vi "Pid_v00.vi"() -> ()   [LabVIEW 2010]
panel:
  in  "stop":bool
  out "u,y,r":cluster{"y":dbl, "u":dbl, "r-Set point":dbl}(graph)={"y"=50.04611274315553, "u"=50.10510244223579, "r-Set point"=50.0}
  in  "Kd":dbl(slide)=0.1151685393258427 scale=0.0..0.5
  in  "Ki":dbl(slide)=0.8764044943820224 scale=0.0..2.0
  in  "Kp":dbl(slide)=0.33707865168539325 scale=0.0..2.5
  out "y-Iesirea":dbl(slide)=50.04611274315553 scale=40.0..60.0
  out "u":dbl(slide)=50.10510244223579 scale=40.0..60.0
  in  "r-Set point":dbl(slide)=50.0 scale=40.0..60.0
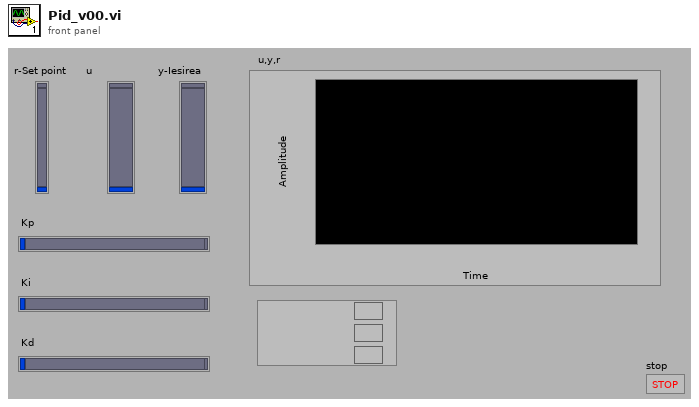
[diagram p1: front panel]
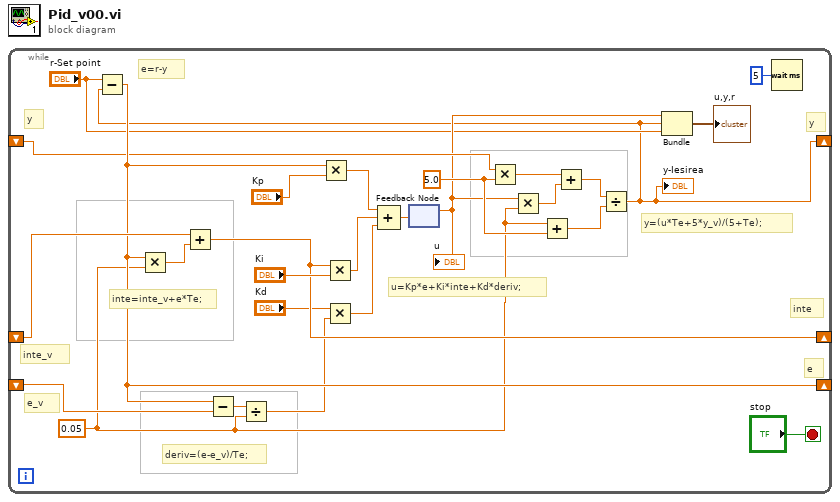
[diagram p0: block diagram]
diagram:
  n1 = while {
    shift-right: [w1] -> _
    shift-left: _ -> [w9]
    shift-right: [w22] -> _
    shift-left: _ -> [w24]
    shift-right: [w17] -> _
    shift-left: _ -> [w18]
    stop <- "stop" stop-if-true
    w7 = 5.0 ("y")
    w6 = 0.05 ("input variable")
    # "e=r-y"
    # "y=(u*Te+5*y_v)/(5+Te);"
    # "u=Kp*e+Ki*inte+Kd*deriv;"
    # "deriv=(e-e_v)/Te;"
    # "inte=inte_v+e*Te;"
    # "e"
    # "inte"
    # "e_v"
    # "inte_v"
    # "y"
    # "y"
    n2 = feedback #1() -> (w4:dbl)  [unwired: 1 in]
    "u" <- w4
    n3 = Multiply(x=w9, y=w7) -> (x*y=w10:dbl)
    n4 = Multiply(x=w4, y=w6) -> (x*y=w8:dbl)
    n5 = Add(x=w6, y=w7) -> (x+y=w11:dbl)
    n6 = Add(x=w10, y=w8) -> (x+y=w12:dbl)
    n7 = Divide(x=w12, y=w11) -> (x/y=w1:dbl)
    "y-Iesirea" <- w1
    n8 = Subtract(x="r-Set point", y=w1) -> (x-y=w17:dbl)
    n9 = Multiply(x=w17, y=w6) -> (x*y=w25:dbl)
    n10 = Add(x=w24, y=w25) -> (x+y=w22:dbl)
    n11 = Subtract(x=w17, y=w18) -> (x-y=w19:dbl)
    n12 = Divide(x=w19, y=w6) -> (x/y=w13:dbl)
    n13 = Multiply(x=w17, y="Kp") -> (x*y=w16:dbl)
    n14 = Multiply(x=w22, y="Ki") -> (x*y=w15:dbl)
    n15 = Multiply(x="Kd", y=w13) -> (x*y=w14:dbl)
    n16 = Compound Arithmetic op=ADD(w16, w15, w14) -> (w5:dbl)
    n17 = feedback-in #1(w5) -> ()
    n18 = Bundle(w4, w1, "r-Set point"="r-Set point") -> (→"u,y,r":cluster{dbl, dbl, "r-Set point":dbl})  [unwired: 1 in]
    n19 = Wait (ms)(milliseconds to wait=u32 5) -> ()  [unwired: 1 out]
  }
